vi "Write Tab Selection Ref.vi"(8 "error in (no error)":errorcluster, 10 "Tab Selection Ref":refnum<vi>, 11 "Settings in":refnum<class "Settings.lvclass">) -> (0 "error out":errorcluster, 3 "Settings out":refnum<class "Settings.lvclass">)   [LabVIEW 2023, in "GUI.lvlib" / "Settings.lvlib" / "Settings.lvclass"]
uses:
  Settings.lvclass
  Settings.lvclass/Settings.ctl
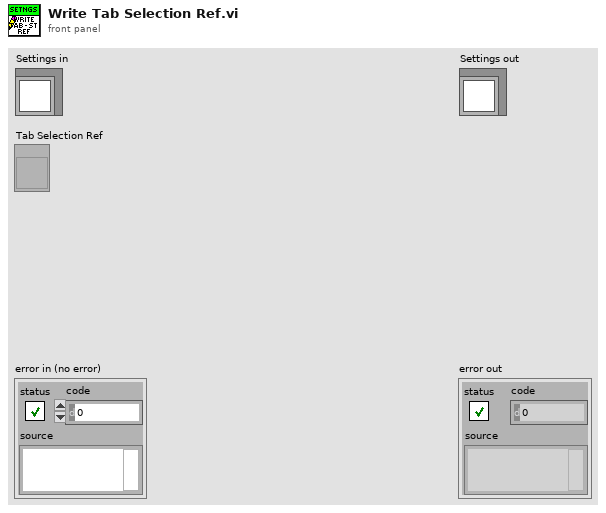
[diagram p1: front panel]
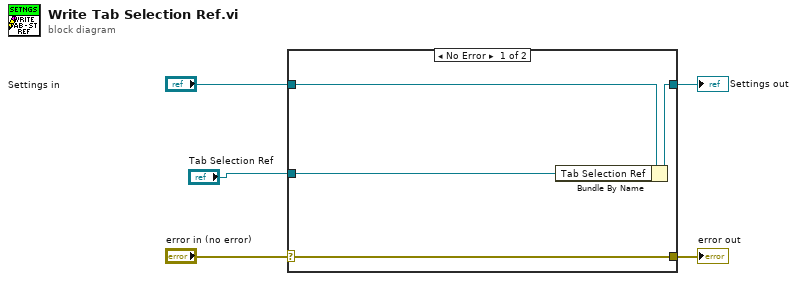
[diagram p0: block diagram]
diagram:
  n1 = case shown="No Error" "error in (no error)" {
    selector: "error in (no error)" -> [w9 w10]
    tunnel: [w9 w10] -> w4
    tunnel: [w7 w11] -> w2
    tunnel: "Settings in" -> [w8 w11]
    tunnel: "Tab Selection Ref" -> [w6 _]
    frame No Error {
      n2 = Bundle By Name(cluster=w8, "Tab Selection Ref"=w6) -> (w7:refnum<class "Settings.lvclass">)
    }
    frame Error {
    }
  }
  "error out" <- w4
  "Settings out" <- w2
